vi "Write U64 FIFO.vi"(0 "input data":u64, 1 "reset":bool, 2 "fifo":refnum<k21>, 9 "input valid":bool) -> (14 "ready for input":bool)   [LabVIEW 2011, in "FIFO.lvlib"]
uses:
  <instrlib>/RF-RIO/FIFO/FIFO/FPGA/FIFO.lvlib
  <vilib>/rvi/DataTransferAndStorage/Container/Common/niFpgaContainerExecOnDevCompGetState.vi
  <vilib>/rvi/FIFO/Fifo_Resource/nirvififoEmulationSetSize.vi
  <vilib>/rvi/DataTransferAndStorage/Container/Common/niFpgaContainerGetUniqueNameForEmu.vi
  <vilib>/rvi/interface/RandomDataEmulation/nirviRandomDataFPGAFIFO.vi
  <vilib>/rvi/interface/RandomDataEmulation/niFpgaRandomDataHandleErrors.vi
  <vilib>/rvi/eio/common/nirviEmuReportErrorAndStop.vi
  <vilib>/rvi/DataTransferAndStorage/Container/XNode/niFpgaContainer.xnode
  <vilib>/rvi/FIFO/Fifo_Resource/niFpgaFifoEmulationRefIn.vi
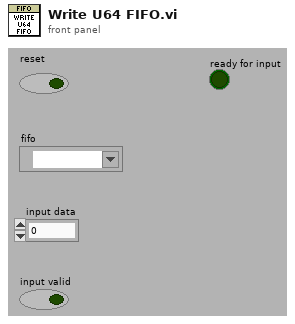
[diagram p1: front panel]
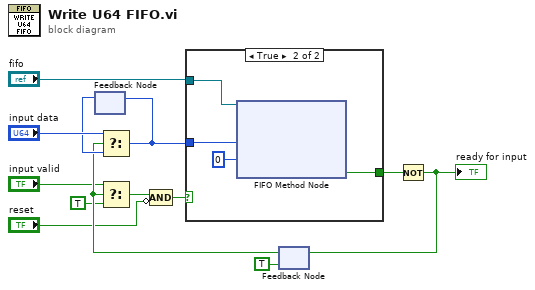
[diagram p0: block diagram]
diagram:
  n1 = feedback #1() -> (w11:u64)  [unwired: 1 in]
  n2 = feedback #2(TRUE) -> (w9:bool)
  n3 = Select(t="input data", s=w9, f=w11) -> (s? t:f=w10:u64)
  n4 = feedback-in #1(w10) -> ()
  n5 = Select(t="input valid", s=w9, f=TRUE) -> (s? t:f=w5:bool)
  n6 = Compound Arithmetic op=AND(w5, invert "reset") -> (w3:bool)
  n7 = case shown="True" w3 {
    tunnel: "fifo" -> [_ w17]
    tunnel: w10 -> [_ w15]
    tunnel: [_ w14] -> w2
    frame False {
    }
    frame True {
      n8 = xnode ("FIFO Method Node")("Element"=w15, "Timeout"=0, "FIFO In"=w17) -> ("Timed Out?"=w14:bool)  [unwired: 1 out]
    }
  }
  n9 = Not(x=w2) -> (.not. x?=w1:bool)
  "ready for input" <- w1
  n10 = feedback-in #2(w1) -> ()
